vi "Init Series.vi"(6 "Series CFG":string, 8 "error in":errorcluster, 9 "Virt Instrs CFG":string, 10 "Instr CFGs":string[](array[string]), 11 "Host MSS Test Actor in":refnum<class "Host MSS Test Actor.lvclass">) -> (0 "error out":errorcluster, 3 "Host MSS Test Actor out":refnum<class "Host MSS Test Actor.lvclass">)   [LabVIEW 2023, in "Host MSS Test Actor.lvlib" / "Host MSS Test Actor.lvclass"]
uses:
  Host MSS Test Actor.lvclass
  C:/Program Files/National Instruments/LabVIEW 2023/vi.lib/ActorFramework/Actor/Actor.lvclass
  Task/Task Actor/Task Actor/Task Actor/Task Actor.lvclass
  <vilib>/ActorFramework/Message Enqueuer/Message Enqueuer.lvclass
  Host MSS Test Actor.lvclass/Host MSS Test Actor.ctl
  Series/Series Base/Series Base.lvclass/Series Base.ctl
  Task/Task Actor/Task Actor/Task Actor/Task Actor.lvclass/Task Actor.ctl
  Series/Series Base/Series Base.lvclass
  <vilib>/ActorFramework/Actor/Actor.lvclass
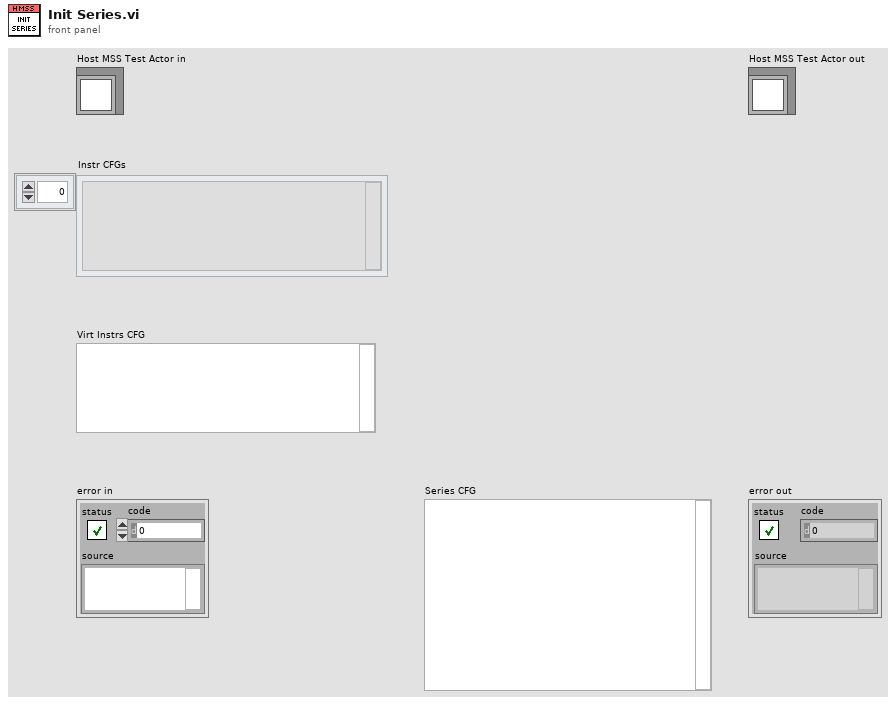
[diagram p1: front panel]
types:
  T1 = map{string, refnum<class "Message Enqueuer.lvclass">}
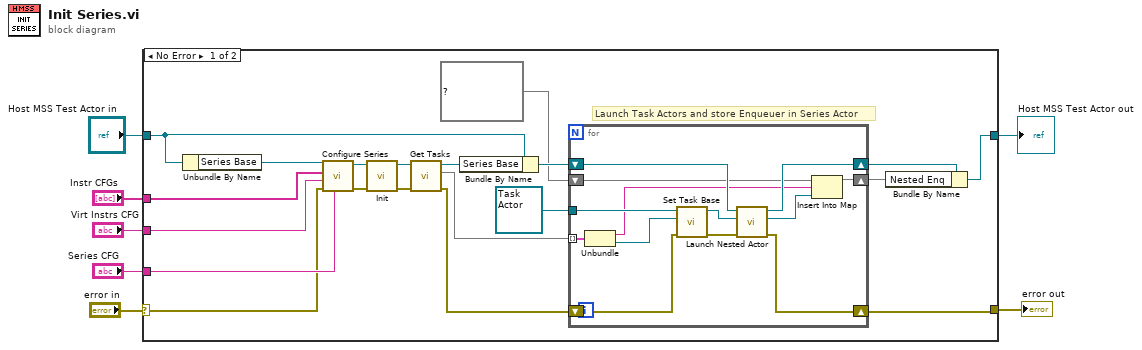
[diagram p0: block diagram]
diagram:
  n1 = case shown="No Error" "error in" {
    selector: "error in" -> [w9 w42]
    tunnel: [w12 w42] -> w6
    tunnel: [w11 w41] -> w4
    tunnel: "Host MSS Test Actor in" -> [w16 w41]
    tunnel: "Instr CFGs" -> [w26 _]
    tunnel: "Virt Instrs CFG" -> [w25 _]
    tunnel: "Series CFG" -> [w24 _]
    frame No Error {
      # "Launch Task Actors and store Enqueuer in Series Actor"
      n2 = Unbundle By Name(w16) -> ("Series Base"=w27:refnum<class "Series Base.lvclass">)
      n3 = call "Configure Series.vi"("Series CFG"=w24, "error in (no error)"=w9, "Virt Instrs CFG"=w25, "Instr CFGs"=w26, "HAL GOOP4:Series Base in"=w27) -> ("error out"=w23:errorcluster, "HAL GOOP4:Series Base out"=w21:refnum<class "Series Base.lvclass">)  [unwired: 5 in]
      n4 = call-dynamic "Init.vi"("error in (no error)"=w23, "HAL GOOP4:Series Base in"=w21) -> ("error out"=w22:errorcluster, "HAL GOOP4:Series Base out"=w20:refnum<class "Series Base.lvclass">)  [unwired: 8 in]
      n5 = call "Get Tasks.vi"("error in (no error)"=w22, "HAL GOOP4:Series Base in"=w20) -> ("error out"=w13:errorcluster, "Tasks"=w18:map{string, refnum<class "Task Base.lvclass">}, "HAL GOOP4:Series Base out"=w19:refnum<class "Series Base.lvclass">)  [unwired: 7 in]
      n6 = Bundle By Name(cluster=w16, "Series Base"=w19) -> (w15:refnum<class "Host MSS Test Actor.lvclass">)
      n7 = for {
        tunnel: w18 -> [w30] mode=indexing
        shift-right: [w34] -> w14
        shift-left: w15 -> [w40]
        tunnel: refnum<class "Task Actor.lvclass"> refnum ("Task Actor.lvlib:Task Actor.lvclass") -> [w39]
        shift-right: [w35] -> w12
        shift-left: w13 -> [w37]
        shift-right: [w32] -> w10
        shift-left: T1 {} ("Size: 0") -> [w33]
        n8 = Unbundle(w30) -> (w29:string, "Task"=w28:refnum<class "Task Base.lvclass">)
        n9 = call "Set Task Base.vi"("error in (no error)"=w37, "HAL GOOP4.lvlib:Task Base.lvclass"=w28, "Task Actor in"=w39) -> ("error out"=w36:errorcluster, "Task Actor out"=w38:refnum<class "Task Actor.lvclass">)  [unwired: 7 in]
        n10 = call <vilib>:"Launch Nested Actor.vi"("error in (no error)"=w36, "Nested Actor"=w38, "Caller Actor in"=w40) -> ("error out"=w35:errorcluster, "Nested Actor's Enqueuer"=w31:refnum<class "Message Enqueuer.lvclass">, "Caller Actor out"=w34:refnum<class "Host MSS Test Actor.lvclass">)  [unwired: 6 in]
        n11 = Insert Into Map(map in=w33, key=w29, value=w31) -> (map out=w32:T1)  [unwired: 2 out]
      }
      n12 = Bundle By Name(cluster=w14, "Nested Enq"=w10) -> (w11:refnum<class "Host MSS Test Actor.lvclass">)
    }
    frame Error {
    }
  }
  "error out" <- w6
  "Host MSS Test Actor out" <- w4
